vi "FPGA_Read_Write.vi"(6 "Motors enabled?":bool, 7 "Reset Encoders?":bool, 9 "Commands":dbl[](array[numeric]), 11 "IO Cluster In":T1={"Error"={"status"=FALSE, "code"=0, "source"=""}, "Encoder Calibration Values"=[22, 216], "Update Calibration"=FALSE, "JPEG Resolutions"=3, "Raw Resolutions"=1, "Image Mode"=enum."RAW Gray Scale", "FPGA Ref"=refnum} {"JPEG Resolutions" items=["160x128"=3, "320x240"=5, "640x480"=7]; "Raw Resolutions" items=["80x60"=1, "160x120"=3, "128x128"=9, "128x96"=11]}) -> (0 "PWM Counts 1":dbl, 1 "Joint Coordinates (rad)":dbl[](array[numeric]), 2 "PWM Counts 0":dbl, 3 "IO Cluster Out":T1={"Error"={"status"=FALSE, "code"=0, "source"=""}, "Encoder Calibration Values"=[22, 216], "Update Calibration"=FALSE, "JPEG Resolutions"=3, "Raw Resolutions"=1, "Image Mode"=enum."RAW Gray Scale", "FPGA Ref"=refnum} {"JPEG Resolutions" items=["160x128"=3, "320x240"=5, "640x480"=7]; "Raw Resolutions" items=["80x60"=1, "160x120"=3, "128x128"=9, "128x96"=11]})   [LabVIEW 2018]
uses:
  QNET MS IO Cluster.ctl
  <vilib>/Utility/error.llb/Error Cluster From Error Code.vi
  <vilib>/rvi/errors/niLvFpgaAdjustHostInterfaceError.vi
  <vilib>/rvi/interface/nirviReadWriteControl/nirviReadWriteControl.xnode
  NiFpgaLv.dll
  <vilib>/rvi/interface/Simulation/niFpgaSimulationCallBeginRW.vi
panel:
  out "PWM Voltages":dbl[](array[numeric])
  out "Stall Error 0":bool
  out "Stall Warning 0":bool
  out "Stall Error 1":bool
  out "Stall Warning 1":bool
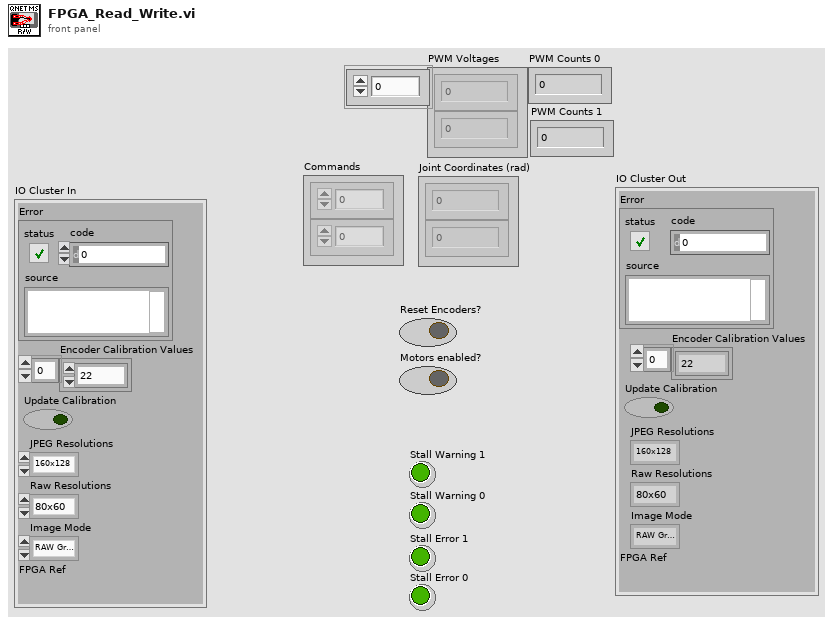
[diagram p1: front panel]
types:
  T1 = typedef "QNET MS IO Cluster.ctl" = cluster{"Error":errorcluster, "Encoder Calibration Values":i32[], "Update Calibration":bool, "JPEG Resolutions":u16, "Raw Resolutions":u16, "Image Mode":enum16{"RAW RGB", "RAW Gray Scale", "JPEG"}, "FPGA Ref":refnum<k20>}
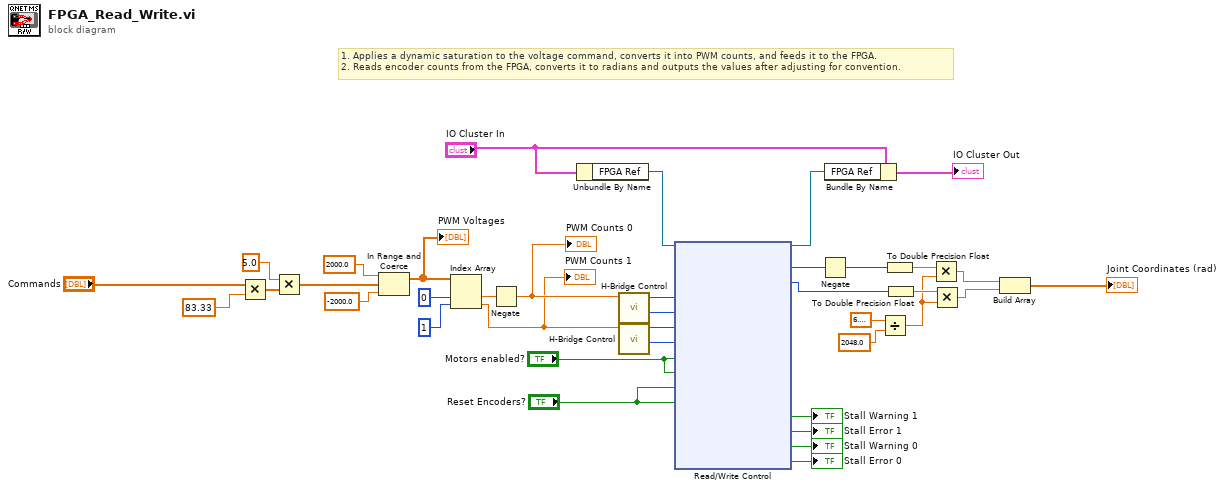
[diagram p0: block diagram]
diagram:
  # "1. Applies a dynamic saturation to the voltage command, converts it into PWM counts, and feeds it to the FPGA.\n2. Reads encoder counts from the FPGA, converts it to radians and outputs the values after adjusting for convention."
  n1 = Multiply(x="Commands", y=83.33) -> (x*y=w21:dbl[])
  n2 = Multiply(x=5.0 ("y"), y=w21) -> (x*y=w9:dbl[])
  n3 = In Range and Coerce(upper limit=2000.0 ("y"), x=w9, lower limit=-2000.0 ("y")) -> (coerced(x)=w8:dbl[])  [unwired: 1 out]
  "PWM Voltages" <- w8
  n4 = Index Array(array=w8, index #1=0 ("index"), index #2=1 ("index 2")) -> (element #1=w7:dbl, element #2=w5:dbl)
  "PWM Counts 1" <- w5
  n5 = Negate(x=w7) -> (-x=w6:dbl)
  "PWM Counts 0" <- w6
  n6 = Unbundle By Name("IO Cluster In") -> ("FPGA Ref"=w17:refnum<k20>)
  n7 = call "H-Bridge Control.vi"("PWM Value (-2000 to 2000)"=w6) -> ("PWM B"=w34:u16, "PWM A"=w37:u16)  [unwired: 9 in]
  n8 = call "H-Bridge Control.vi"("PWM Value (-2000 to 2000)"=w5) -> ("PWM B"=w36:u16, "PWM A"=w35:u16)  [unwired: 9 in]
  n9 = xnode ("Read/Write Control")("FPGA VI Reference In"=w17, "PWM.0A"=w37, "PWM.0B"=w34, "PWM.1A"=w35, "PWM.1B"=w36, "PWM0 Enable"="Motors enabled?", "PWM1 Enable"="Motors enabled?", "Encoder 0 Reset"="Reset Encoders?", "Encoder 1 Reset"="Reset Encoders?") -> ("FPGA VI Reference Out"=w16:refnum<k20>, "Encoder 0 Counter"=w4:i32, "Encoder 1 Counter"=w2:i32, "Stall Warning 1"=→"Stall Warning 1":bool, "Stall Error 1"=→"Stall Error 1":bool, "Stall Warning 0"=→"Stall Warning 0":bool, "Stall Error 0"=→"Stall Error 0":bool)  [unwired: 1 in, 1 out]
  n10 = Negate(x=w4) -> (-x=w3:i32)
  n11 = Bundle By Name(cluster="IO Cluster In", "FPGA Ref"=w16) -> (→"IO Cluster Out":T1)
  n12 = Divide(x=6.283185307179586 ("Constant 2"), y=2048.0) -> (x/y=w24:dbl)
  n13 = To Double Precision Float(number=w3) -> (double precision float=w27:dbl)
  n14 = To Double Precision Float ("To Double Precision Float 2")(number=w2) -> (double precision float=w28:dbl)
  n15 = Multiply(x=w27, y=w24) -> (x*y=w20:dbl)
  n16 = Multiply ("Multiply 2")(x=w28, y=w24) -> (x*y=w19:dbl)
  n17 = Build Array(w20, w19) -> (→"Joint Coordinates (rad)":dbl[])
